vi "EncodeCommand.vi"(0 "Address":string="X", 1 "Function":string, 7 "Data":string) -> (4 "Command String":string, 6 "Command":i32[](array[numeric]))   [LabVIEW 2020, in "Reader.lvlib"]
uses:
  UART/Reader.lvlib
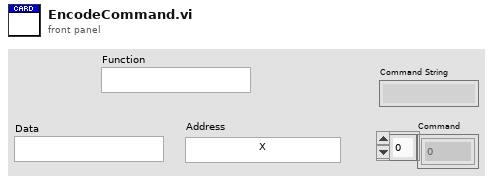
[diagram p1: front panel]
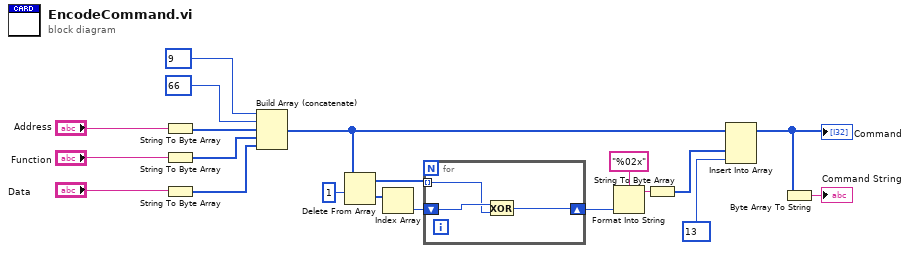
[diagram p0: block diagram]
diagram:
  n1 = String To Byte Array(string="Address") -> (unsigned byte array=w9:u8[])
  n2 = String To Byte Array(string="Function") -> (unsigned byte array=w7:u8[])
  n3 = String To Byte Array(string="Data") -> (unsigned byte array=w6:u8[])
  n4 = Build Array (concatenate)(9, 66, w9, w7, w6) -> (w5:i32[])
  n5 = Delete From Array(array=w5, length=1) -> (deleted portion=w17:i32[], array with subset deleted=w18:i32[])  [unwired: 1 in]
  n6 = Index Array(array=w17) -> (element=w16:i32)  [unwired: 1 in]
  n7 = for {
    tunnel: w18 -> [w21] mode=indexing
    shift-right: [w23] -> w15
    shift-left: w16 -> [w22]
    n8 = Exclusive Or(1:w21, 2:w22) -> (0:w23:i32)
  }
  n9 = Format Into String(format string="%02x", w15) -> (resulting string=w13:string)  [unwired: 2 in, 1 out]
  n10 = String To Byte Array(string=w13) -> (unsigned byte array=w20:u8[])
  n11 = Insert Into Array(array=w5, new element #1=w20, new element #2=13) -> (w3:i32[])  [unwired: 1 in]
  "Command" <- w3
  n12 = Byte Array To String(unsigned byte array=w3) -> (string=→"Command String":string)
